vi "TDC_DAQV_CountingRate_muon.vi"(7 "bytes to read":i32=1600, 9 "UDP Config":bool=TRUE, 10 "timeout":dbl=4500.0) -> (0 "error out":errorcluster, 1 "pmt_trigger_rate":dbl[](array[numeric])=[10.0, 4.0, 3.0, 6.0, 13.0, 7.0, 32615.0, 19574.0, 42.0, 11.0, 6.0, 40.0, 20.0, 5.0, 17.0, 21.0, 8.0, 5054.0, 15.0, 837.0, 5.0, 12.0, 0.0, 30.0, 23040.0, 1.0, 7.0, 57773.0, 4.0, 6.0, 15.0, 10.0, 7.0, 2.0, 7.0, 25615.0, 32.0, 54486.0, 5.0, 6.0, 2716.0, 28.0, 4.0, 8.0, 17.0, 17605.0, 8.0, 5695.0, 6.0, 0.0], 2 "time":dbl=450.0011610984802, 3 "rate":dbl=26781.661574353802)   [LabVIEW 2017]
panel:
  out "无符号字节数组":u8[](array[numeric])
  out "Out 2":u8 format="%.0x"
  in  "Array":string[](array[string])=["192.168.10.20"]
  in  "Thresholds":dbl=-0.03
  in  "one key for threshold":bool=TRUE
  out "DAC":dbl=8094.0
  in  "SMA mode":bool
  in  "Thresholds (mV)":dbl[](array[numeric])=[580.0, 580.0, 580.0, 580.0, 600.0, 600.0, 600.0, 600.0, 580.0, 580.0, 600.0, 600.0, 600.0, 600.0, 600.0, 600.0, 580.0, 580.0, 600.0, 600.0, 600.0, 600.0, 600.0, 600.0, 580.0, 580.0, 600.0, 600.0, 600.0, 600.0, 600.0, 600.0, 600.0, 600.0, 600.0, 600.0, 600.0, 600.0, 600.0, 600.0, 600.0, 600.0, 600.0, 600.0, 600.0, 600.0, 600.0, 600.0, 600.0, 600.0, 600.0, 600.0, 600.0, 600.0, 600.0, 600.0, 600.0, 600.0, 600.0, 600.0, 600.0, 600.0, 600.0, 600.0]
  out "Out":u8=3 format="%.0x"
  in  "error in (no error)":errorcluster
  out "rate_array 2":dbl[](array[numeric])=[10.0, 0.0, 4.0, 0.0, 3.0, 0.0, 6.0, 0.0, 13.0, 0.0, 7.0, 0.0, 32615.0, 0.0, 19574.0, 0.0, 42.0, 0.0, 11.0, 0.0, 6.0, 0.0, 40.0, 0.0, 20.0, 0.0, 5.0, 0.0, 17.0, 0.0, 21.0, 0.0, 8.0, 0.0, 5054.0, 0.0, 15.0, 0.0, 837.0, 0.0, 5.0, 0.0, 12.0, 0.0, 0.0, 0.0, 30.0, 0.0, 23040.0, 23040.0, 1.0, 0.0, 7.0, 0.0, 57773.0, 0.0, 4.0, 0.0, 6.0, 0.0, 15.0, 0.0, 10.0, 0.0, 7.0, 0.0, 2.0, 0.0, 7.0, 0.0, 25615.0, 0.0, 32.0, 0.0, 54486.0, 0.0, 5.0, 0.0, 6.0, 0.0, 2716.0, 0.0, 28.0, 0.0, 4.0, 0.0, 8.0, 0.0, 17.0, 0.0, 17605.0, 0.0, 8.0, 0.0, 5695.0, 0.0, 6.0, 0.0, 0.0, 0.0]
  out "数值":dbl=50.0
  out "sent number 2":u64=19574 format="%x"
  out "data 9":string
  out "sent number":u64=3660 format="%x"
  out "substring 2":string
  out "channel number":u64=14 format="%x"
  out "substring":string
  out "array":dbl[](array[numeric])=[-1.0, -1.0, -1.0, -1.0, -1.0, -1.0, -1.0, -1.0, -1.0, -1.0, -1.0, -1.0, -1.0, -1.0, -1.0, -1.0, -1.0, -1.0, -1.0, -1.0, -1.0, -1.0, -1.0, -1.0, -1.0, -1.0, -1.0, -1.0, -1.0, -1.0, -1.0, -1.0, -1.0, -1.0, -1.0, -1.0, -1.0, -1.0, -1.0, -1.0, -1.0, -1.0, -1.0, -1.0, -1.0, -1.0, -1.0, -1.0, -1.0, -1.0, -1.0, -1.0, -1.0, -1.0, -1.0, -1.0, -1.0, -1.0, -1.0, -1.0, -1.0, -1.0, -1.0, -1.0, -1.0, -1.0, -1.0, -1.0, -1.0, -1.0, -1.0, -1.0, -1.0, -1.0, -1.0, -1.0, -1.0, -1.0, -1.0, -1.0, -1.0, -1.0, -1.0, -1.0, -1.0, -1.0, -1.0, -1.0, -1.0, -1.0, -1.0, -1.0, -1.0, -1.0, -1.0, -1.0, -1.0, -1.0, -1.0, -1.0]
  out "trigger number":u64=19574 format="%x"
  out "data 8":string="Lv"
  out "concatenated string":string
  out "number":u32=20
  in  "factor":i32=2
  in  "stop":bool
  in  "timeout (ms)":i32=8400
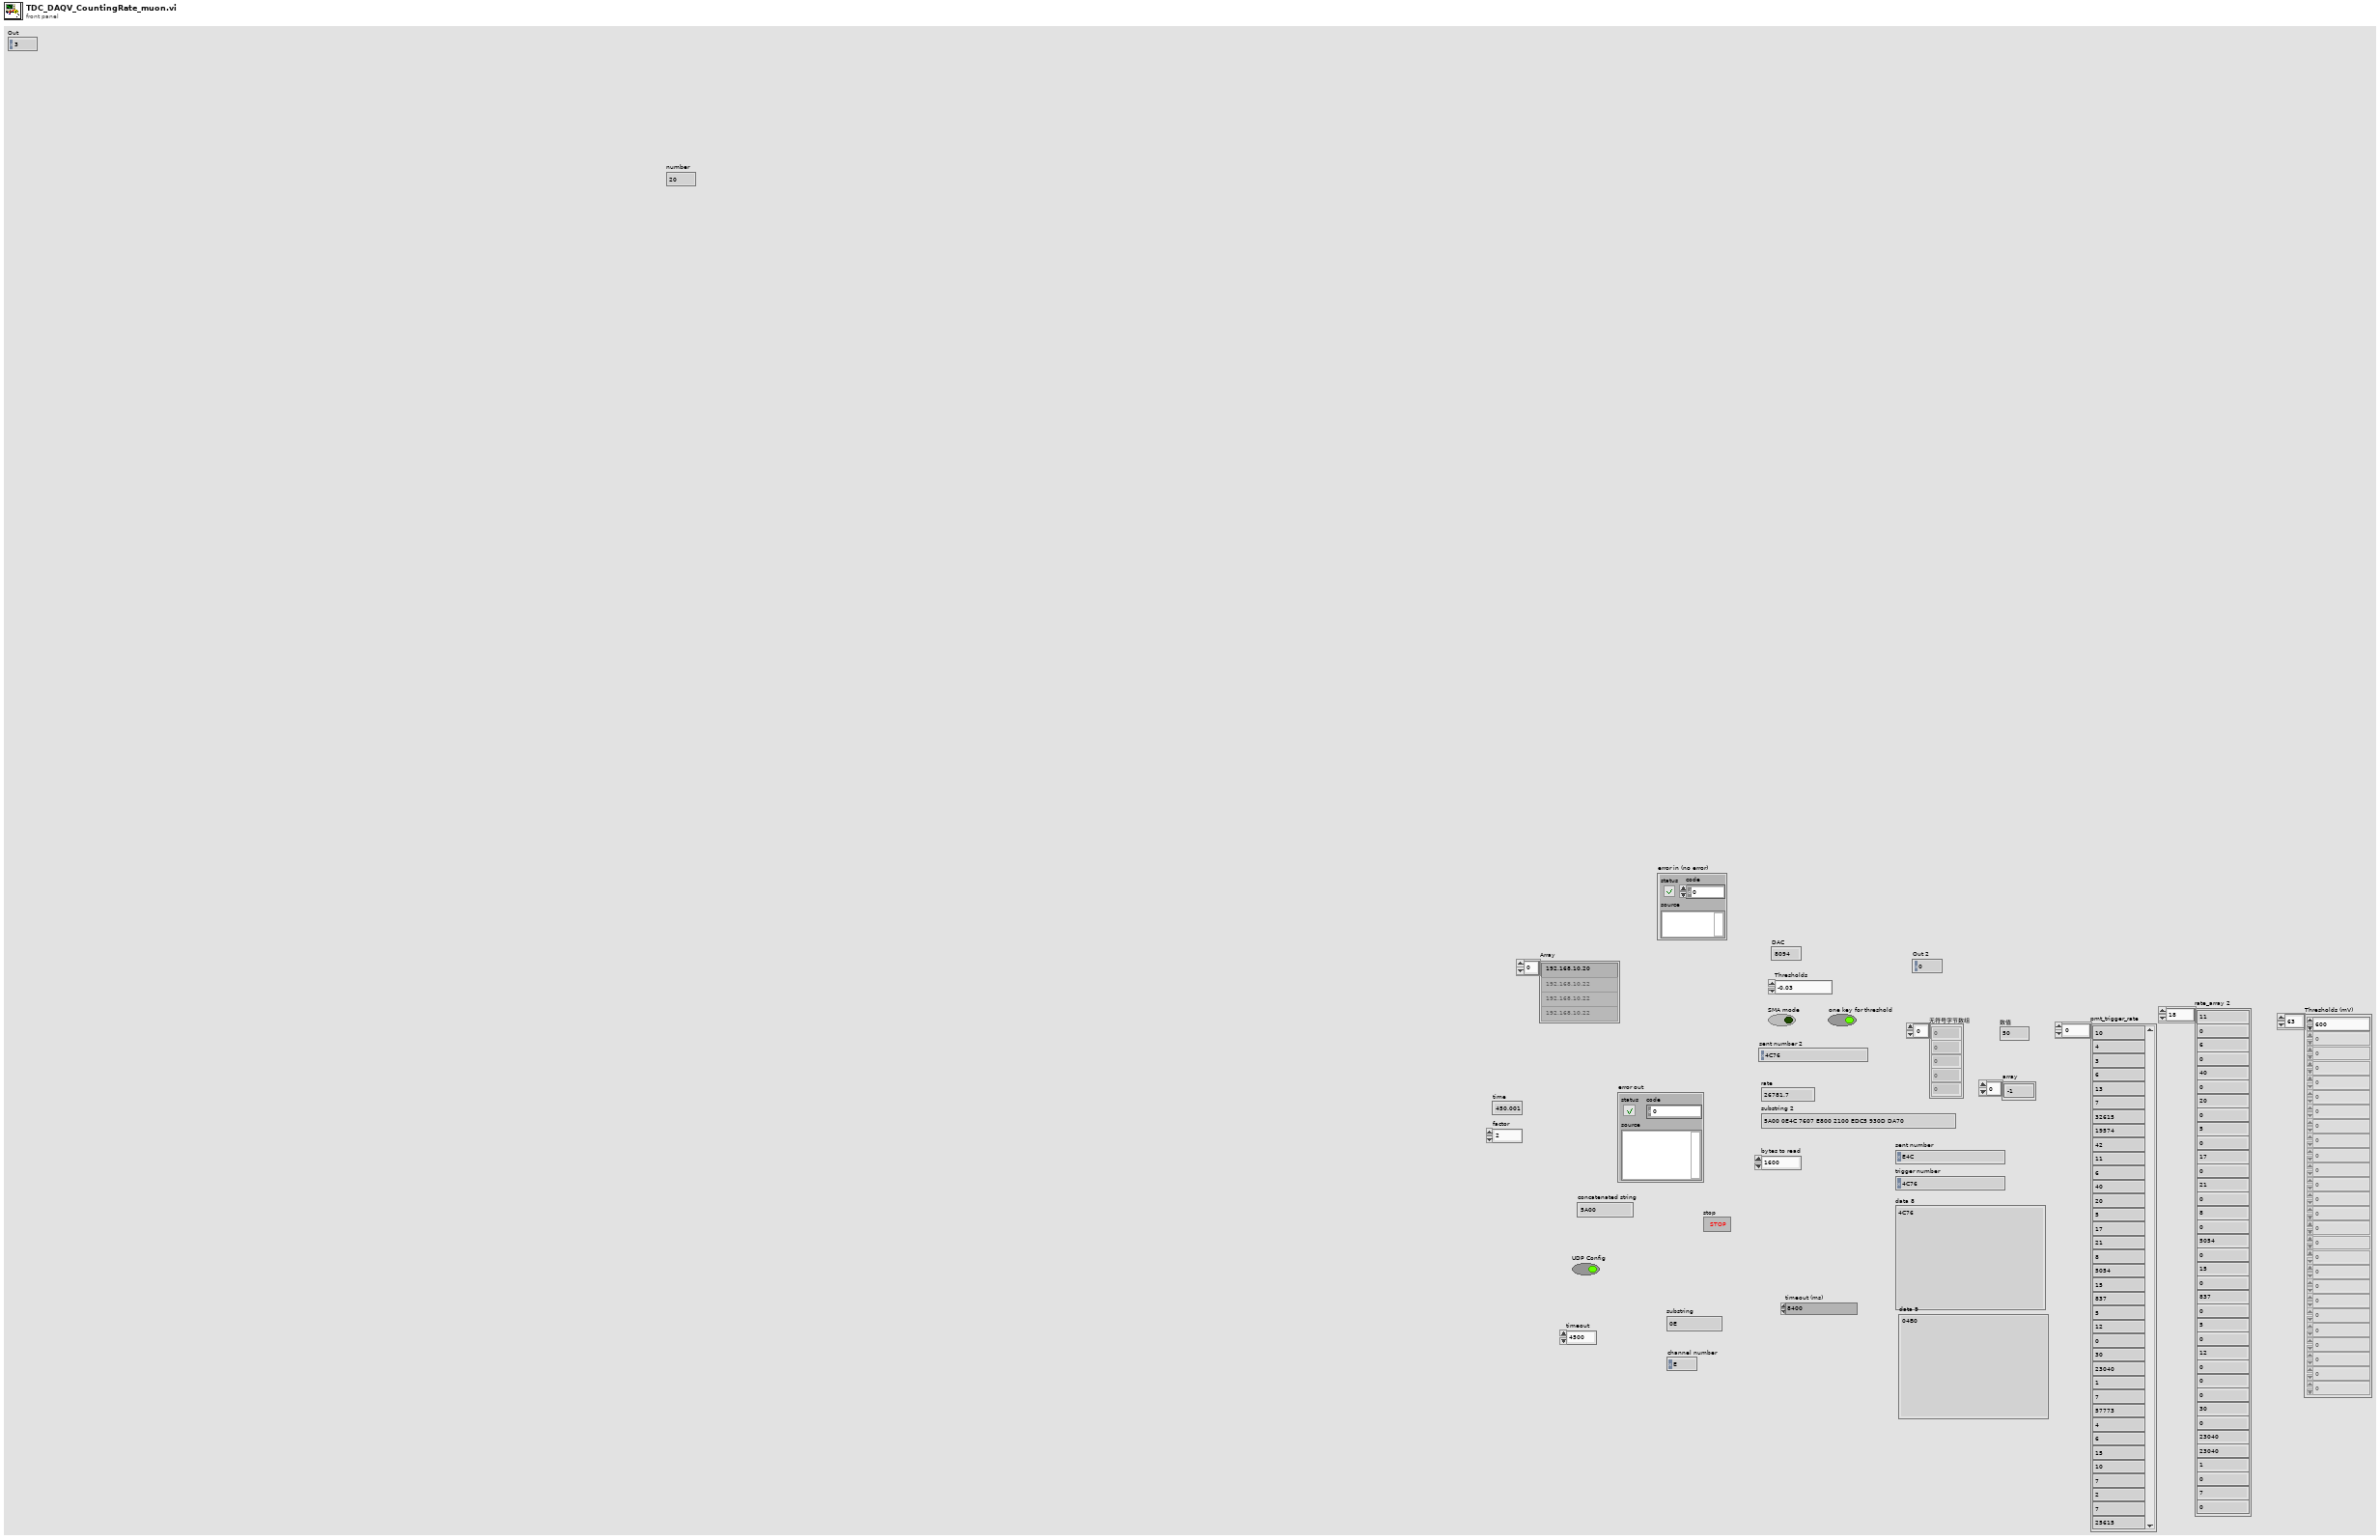
[diagram p1: front panel]
types:
  T1 = enum16{"Standard", "Buffered", "CRLF", "Immediate"}
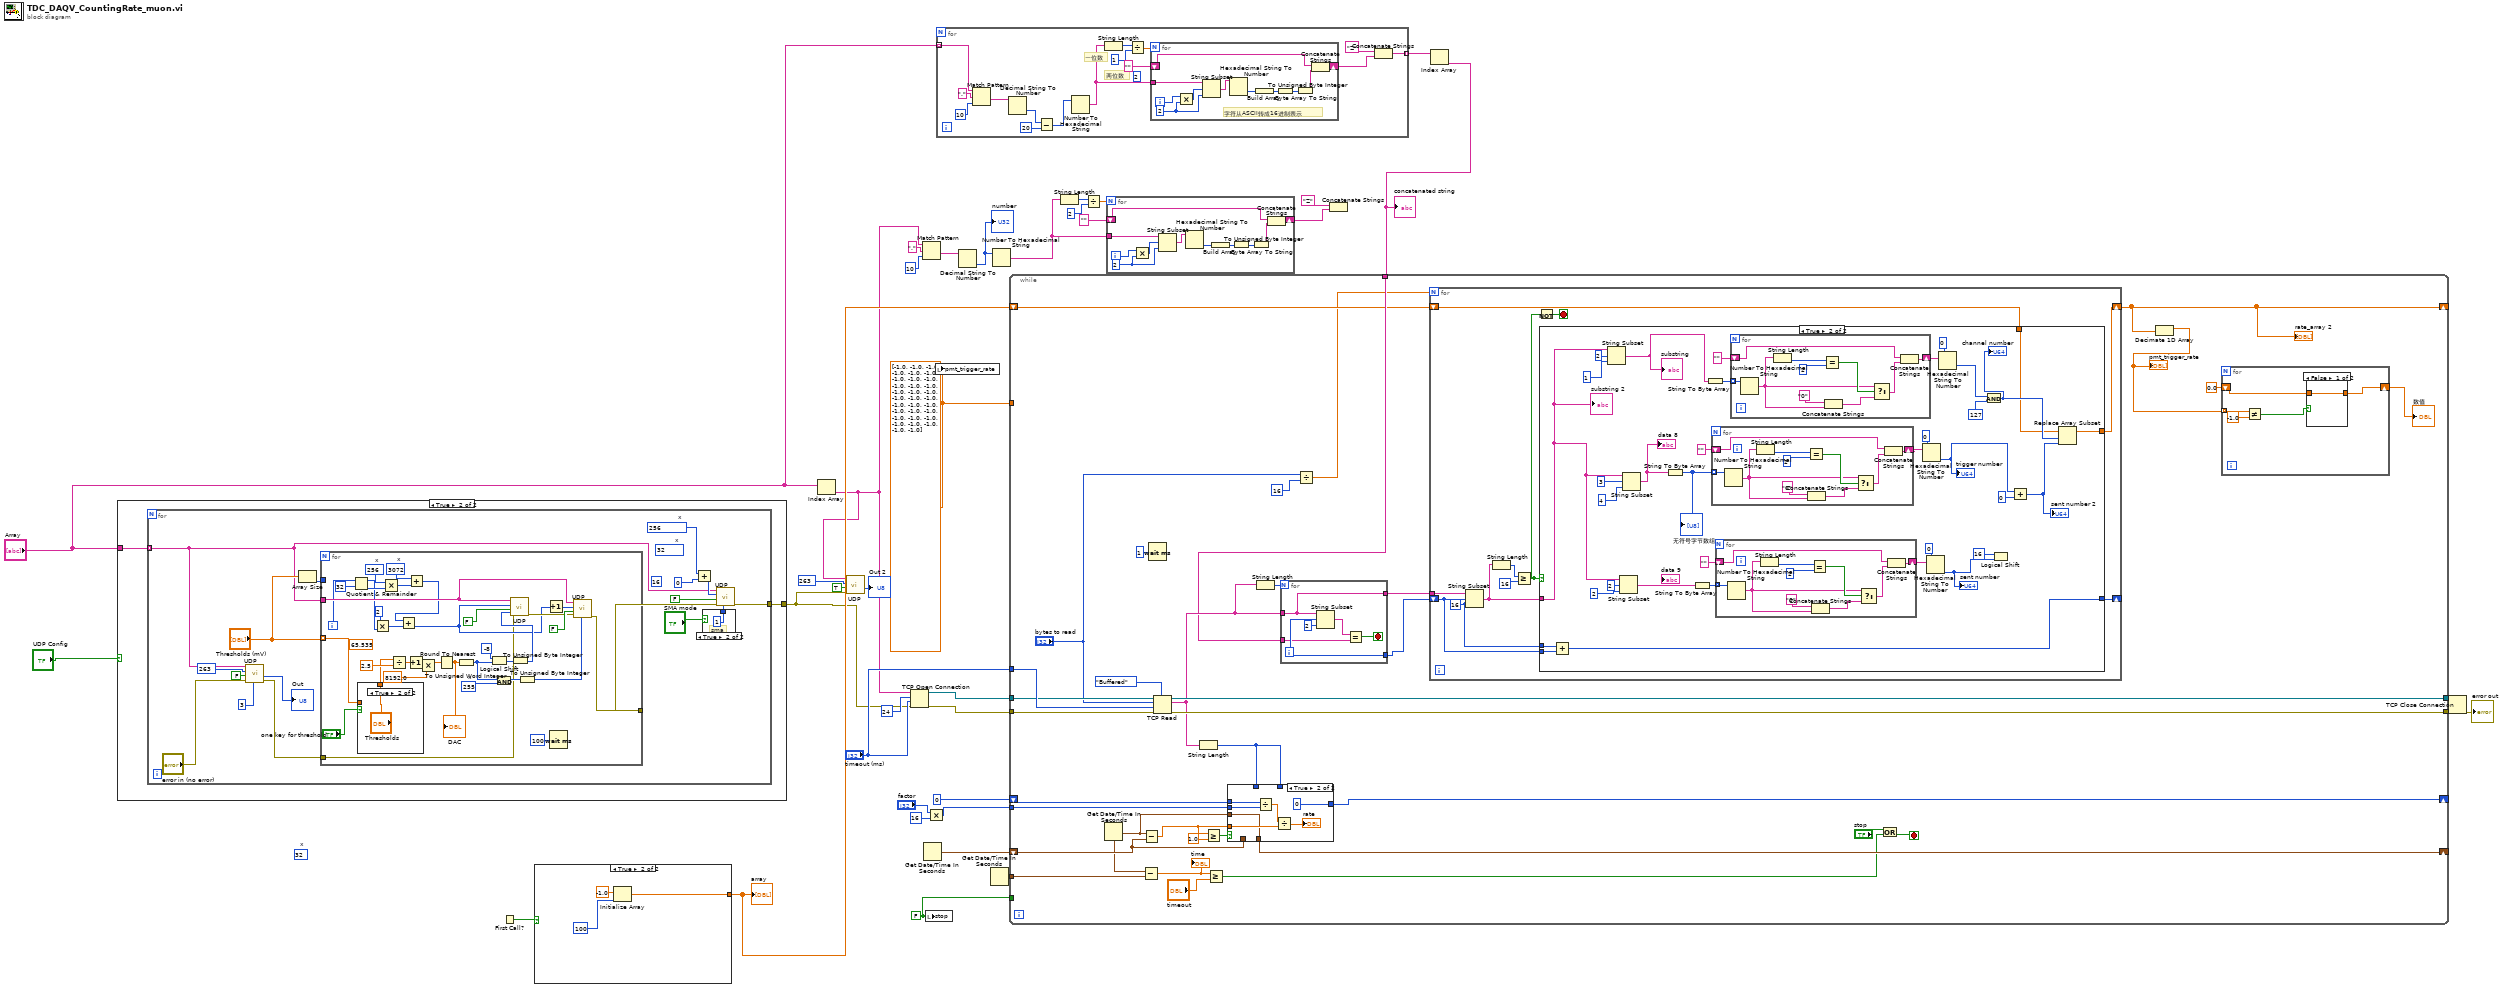
[diagram p0: block diagram]
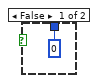
[diagram p3: hidden frame]
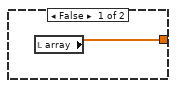
[diagram p5: hidden frame]
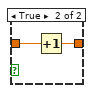
[diagram p6: hidden frame]
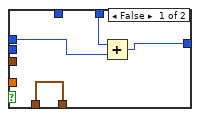
[diagram p8: hidden frame]
diagram:
  w10 = dbl[] [-1.0, -1.0, -1.0, -1.0, -1.0, -1.0, -1.0, -1.0, -1.0, -1.0, -1.0, -1.0, -1.0, -1.0, -1.0, -1.0, -1.0, -1.0, -1.0, -1.0, -1.0, -1.0, -1.0, -1.0, -1.0, -1.0, -1.0, -1.0, -1.0, -1.0, -1.0, -1.0] ("rate_array")
  w25 = FALSE ("stop")
  (unwired) u16 32  # x
  n1 = case shown="True" "UDP Config" {
    tunnel: "Array" -> [_ w38]
    tunnel: [_ w39] -> w3
    frame False {
    }
    frame True {
      n2 = for {
        tunnel: [w54] -> w39
        tunnel: w38 -> [w42] mode=indexing
        (unwired) u16 32  # x
        (unwired) u32 16 ("Address")
        w47 = u16 256  # x
        n3 = call "UDP.vi"("In"=u8 3, "error in (no error)"="error in (no error)", "Read (TRUE)"=FALSE, "Address"=u32 263, "IP address"=w42) -> ("error out"=w40:errorcluster, "Out"=→"Out":u8)  [unwired: 3 in, 1 out]
        n4 = Array Size(array="Thresholds (mV)") -> (size(s)=w51:i32)
        n5 = for {
          tunnel: w42 -> [w88]
          tunnel: "Thresholds (mV)" -> [w75] mode=indexing
          tunnel: [w78] -> w55
          tunnel: w51 -> [_]
          tunnel: w40 -> [w62]
          i -> [w70]
          (unwired) 65.535 ("y")
          w71 = u16 3072  # x
          w72 = u16 256  # x
          w84 = u16 255  # x
          n6 = Quotient & Remainder(x=w70, y=32) -> (x-y*floor(x/y)=w64:i32, floor(x/y)=w73:i32)
          n7 = case shown="True" "one key for threshold" {
            tunnel: [w94 "Thresholds"] -> w76
            tunnel: w75 -> [w94 _]
            frame False {
            }
            frame True {
            }
          }
          n8 = Multiply(x=2, y=w64) -> (x*y=w65:i32)
          n9 = Multiply(x=w72, y=w73) -> (x*y=w67:i32)
          n10 = Divide(x=w76, y=2.5) -> (x/y=w91:dbl)
          n11 = Increment(x=w91) -> (x+1=w61:dbl)
          n12 = Add(x=w71, y=w67) -> (x+y=w66:i32)
          n13 = Add(x=w66, y=w65) -> (x+y=w69:i32)
          n14 = Multiply(x=w61, y=8192.0) -> (x*y=w60:dbl)
          n15 = Round To Nearest(number=w60) -> (nearest integer value=w89:dbl)
          "DAC" <- w89
          n16 = To Unsigned Word Integer(number=w89) -> (unsigned 16bit integer=w80:u16)
          n17 = Logical Shift(y=i16 -8, x=w80) -> (x << y=w86:u16)
          n18 = And(x=w80, y=w84) -> (x .and. y?=w83:u16)
          n19 = To Unsigned Byte Integer(number=w86) -> (unsigned 8bit integer=w85:u8)
          n20 = call "UDP.vi"("In"=w85, "error in (no error)"=w62, "Read (TRUE)"=FALSE, "Address"=w69, "IP address"=w88) -> ("error out"=w79:errorcluster)  [unwired: 3 in, 2 out]
          n21 = To Unsigned Byte Integer(number=w83) -> (unsigned 8bit integer=w82:u8)
          n22 = Increment(x=w69) -> (x+1=w68:i32)
          n23 = Wait (ms)(milliseconds to wait=u32 100) -> ()  [unwired: 1 out]
          n24 = call "UDP.vi"("In"=w82, "error in (no error)"=w79, "Read (TRUE)"=FALSE, "Address"=w68, "IP address"=w88) -> ("error out"=w78:errorcluster)  [unwired: 3 in, 2 out]
        }
        n25 = Add(x=w47, y=u32 0 ("Address")) -> (x+y=w48:u32)
        n26 = case shown="True" "SMA mode" {
          tunnel: [u8 0 ("In") u8 1 ("In")] -> w53
          frame False {
          }
          frame True {
            # "sma"
          }
        }
        n27 = call "UDP.vi"("In"=w53, "error in (no error)"=w55, "Read (TRUE)"=FALSE, "Address"=w48, "IP address"=w42) -> ("error out"=w54:errorcluster)  [unwired: 3 in, 2 out]
      }
    }
  }
  n28 = First Call?() -> (First Call?: T/F=w12:bool)
  n29 = case shown="True" w12 {
    tunnel: [w96 w97] -> w11
    frame False {
      n30 = local read "array"() -> (w96:dbl[])
    }
    frame True {
      n31 = Initialize Array(-1.0 ("element"), 100 ("dimension size")) -> (w97:dbl[])
    }
  }
  "array" <- w11
  n32 = Index Array(array="Array") -> (element=w2:string)  [unwired: 1 in]
  n33 = call "UDP.vi"("error in (no error)"=w3, "Read (TRUE)"=TRUE, "Address"=u32 263, "IP address"=w2) -> ("Out"=→"Out 2":u8)  [unwired: 4 in, 2 out]
  n34 = TCP Open Connection(address=w2, remote port or service name=u16 24 ("port"), timeout ms (60000)="timeout (ms)", error in (no error)=w3) -> (connection ID=w35:refnum<k5>, error out=w36:errorcluster)  [unwired: 1 in]
  n35 = Match Pattern(string=w2, regular expression="." ("search string"), offset (0)=10) -> (after substring=w16:string)  [unwired: 3 out]
  n36 = Get Date/Time In Seconds() -> (seconds since 1Jan1904=w31:timestamp)
  n37 = local write "stop"(w25) -> ()
  n38 = Multiply(x="factor", y=16) -> (x*y=w27:i32)
  n39 = local write "pmt_trigger_rate"(w10) -> ()
  n40 = for {
    tunnel: [w101] -> w7 mode=indexing
    tunnel: "Array" -> [w100] mode=indexing
    (unwired) 2 ("y")
    # "一位数"
    # "两位数"
    n41 = Match Pattern(string=w100, regular expression="." ("search string"), offset (0)=10) -> (after substring=w107:string)  [unwired: 3 out]
    n42 = Decimal String To Number(string=w107) -> (number=w104:i32)  [unwired: 2 in, 1 out]
    n43 = Subtract(x=w104, y=20) -> (x-y=w103:i32)
    n44 = Number To Hexadecimal String(2:w103) -> (0:w106:string)  [unwired: 1 in]
    n45 = String Length(string=w106) -> (length=w112:i32)
    n46 = Divide(x=w112, y=1) -> (x/y=w113:dbl)
    n47 = for {
      N: w113 -> [_]
      shift-right: [w125] -> w102
      shift-left: "" ("format string") -> [w124]
      tunnel: w106 -> [w115]
      i -> [w123]
      w117 = 2 ("y")
      # "字符从ASCII转成16进制表示"
      n48 = Multiply(x=w123, y=w117) -> (x*y=w116:i32)
      n49 = String Subset(string=w115, offset (0)=w116, length (rest)=w117) -> (substring=w118:string)
      n50 = Hexadecimal String To Number(string=w118) -> (number=w122:u32)  [unwired: 2 in, 1 out]
      n51 = Build Array(w122) -> (w121:u32[])
      n52 = To Unsigned Byte Integer(number=w121) -> (unsigned 8bit integer=w120:u8[])
      n53 = Byte Array To String(unsigned byte array=w120) -> (string=w119:string)
      n54 = Concatenate Strings(w124, w119) -> (w125:string)
    }
    n55 = Concatenate Strings("Z", w102) -> (w101:string)
  }
  n56 = Decimal String To Number(string=w16) -> (number=w15:i32)  [unwired: 2 in, 1 out]
  "number" <- w15
  n57 = Get Date/Time In Seconds() -> (seconds since 1Jan1904=w24:timestamp)
  n58 = Number To Hexadecimal String(2:w15) -> (0:w14:string)  [unwired: 1 in]
  n59 = String Length(string=w14) -> (length=w21:i32)
  n60 = Divide(x=w21, y=2) -> (x/y=w22:dbl)
  n61 = for {
    N: w22 -> [_]
    shift-right: [w136] -> w13
    shift-left: "" ("format string") -> [w135]
    tunnel: w14 -> [w126]
    i -> [w134]
    w128 = 2 ("y")
    n62 = Multiply(x=w134, y=w128) -> (x*y=w127:i32)
    n63 = String Subset(string=w126, offset (0)=w127, length (rest)=w128) -> (substring=w129:string)
    n64 = Hexadecimal String To Number(string=w129) -> (number=w133:u32)  [unwired: 2 in, 1 out]
    n65 = Build Array(w133) -> (w132:u32[])
    n66 = To Unsigned Byte Integer(number=w132) -> (unsigned 8bit integer=w131:u8[])
    n67 = Byte Array To String(unsigned byte array=w131) -> (string=w130:string)
    n68 = Concatenate Strings(w135, w130) -> (w136:string)
  }
  n69 = Concatenate Strings("Z", w13) -> ()  [unwired: 1 out]
  n70 = Index Array(array=w7) -> (element=w6:string)  [unwired: 1 in]
  "concatenated string" <- w6
  n71 = while {
    tunnel: w36 -> [w172]
    tunnel: "timeout (ms)" -> [w171]
    tunnel: w35 -> [w170]
    tunnel: [w169] -> w34
    tunnel: [w168] -> w33
    shift-right: [w161] -> _
    shift-left: w31 -> [w165]
    shift-right: [w164] -> _
    shift-left: u32 0 ("milliseconds to wait") -> [w159]
    tunnel: w27 -> [w158]
    tunnel: w25 -> [_]
    tunnel: w24 -> [w152]
    tunnel: w6 -> [w146]
    shift-right: [w137] -> _
    shift-left: w11 -> [w145]
    tunnel: w10 -> [_]
    stop <- w155 stop-if-true
    n72 = Get Date/Time In Seconds() -> (seconds since 1Jan1904=w151:timestamp)
    n73 = Subtract(x=w151, y=w152) -> (x-y=w150:dbl)
    "time" <- w150
    n74 = Subtract(x=w151, y=w165) -> (x-y=w157:dbl)
    n75 = Wait (ms)(milliseconds to wait=u32 1) -> ()  [unwired: 1 out]
    n76 = TCP Read(connection ID=w170, bytes to read="bytes to read", error in (no error)=w172, 7:T1."Buffered" ("mode (standard)"), 9:w171) -> (connection ID out=w169:refnum<k5>, data out=w147:string, error out=w168:errorcluster)
    n77 = String Length(string=w147) -> (length=w160:i32)
    n78 = Greater Or Equal?(x=w157, y=1.0) -> (x >= y?=w163:bool)
    n79 = Greater Or Equal?(x=w150, y="timeout") -> (x >= y?=w153:bool)
    n80 = case shown="True" w163 {
      tunnel: w157 -> [_ w275]
      tunnel: w151 -> [_ w273]
      tunnel: [w268 w273] -> w161
      tunnel: w165 -> [w268 _]
      tunnel: w160 -> [_ _]
      tunnel: w160 -> [w267 _]
      tunnel: [w266 0] -> w164
      tunnel: w158 -> [_ w270]
      tunnel: w159 -> [w265 w269]
      frame False {
        n81 = Add(x=w267, y=w265) -> (x+y=w266:u32)
      }
      frame True {
        n82 = Divide(x=w269, y=w270) -> (x/y=w272:dbl)
        n83 = Divide(x=w272, y=w275) -> (x/y=→"rate":dbl)
      }
    }
    n84 = String Length(string=w147) -> (length=w149:i32)
    n85 = for {
      N: w149 -> [_]
      tunnel: w147 -> [w261]
      tunnel: [w261] -> w148
      tunnel: [w260] -> w144
      tunnel: w146 -> [w259]
      i -> [w260]
      stop <- w262 stop-if-true
      n86 = String Subset(string=w261, offset (0)=w260, length (rest)=2 ("length (rest)")) -> (substring=w263:string)
      n87 = Equal?(x=w263, y=w259) -> (x = y?=w262:bool)
    }
    n88 = Divide(x="bytes to read", y=16 ("length (rest)")) -> (x/y=w141:dbl)
    n89 = for {
      N: w141 -> [_]
      tunnel: w148 -> [w191]
      shift-right: [w189] -> w137
      shift-left: w145 -> [w190]
      shift-right: [w181] -> _
      shift-left: w144 -> [w182]
      stop <- w184 stop-if-true
      w183 = 16 ("length (rest)")
      n90 = String Subset(string=w191, offset (0)=w182, length (rest)=w183) -> (substring=w188:string)
      n91 = String Length(string=w188) -> (length=w187:i32)
      n92 = Greater Or Equal?(x=w187, y=16 ("length (rest)")) -> (x >= y?=w185:bool)
      n93 = Not(x=w185) -> (.not. x?=w184:bool)
      n94 = case shown="True" w185 {
        tunnel: w188 -> [_ w209]
        tunnel: w190 -> [w193 w208]
        tunnel: [w193 w207] -> w189
        tunnel: w182 -> [w192 w206]
        tunnel: w183 -> [_ w205]
        tunnel: [w192 w204] -> w181
        frame False {
        }
        frame True {
          n95 = Add(x=w205, y=w206) -> (x+y=w204:i32)
          n96 = String Subset(string=w209, offset (0)=2, length (rest)=1 ("length (rest)")) -> (substring=w213:string)
          "substring" <- w213
          n97 = String Subset(string=w209, offset (0)=2, length (rest)=2 ("length (rest)")) -> (substring=w199:string)
          n98 = String Subset(string=w209, offset (0)=3, length (rest)=4 ("length (rest)")) -> (substring=w220:string)
          "data 8" <- w220
          n99 = String To Byte Array(string=w220) -> (unsigned byte array=w222:u8[])
          "无符号字节数组" <- w222
          n100 = String To Byte Array(string=w199) -> (unsigned byte array=w202:u8[])
          n101 = String To Byte Array(string=w213) -> (unsigned byte array=w216:u8[])
          n102 = for {
            shift-right: [w257] -> w223
            shift-left: "" ("format string") -> [w254]
            tunnel: w222 -> [w258] mode=indexing
            n103 = Number To Hexadecimal String(2:w258) -> (0:w250:string)  [unwired: 1 in]
            n104 = String Length(string=w250) -> (length=w256:i32)
            n105 = Equal?(x=w256, y=2) -> (x = y?=w253:bool)
            n106 = Concatenate Strings("0" ("format string"), w250) -> (w252:string)
            n107 = Select(t=w250, s=w253, f=w252) -> (s? t:f=w249:string)
            n108 = Concatenate Strings(w254, w249) -> (w257:string)
          }
          n109 = for {
            shift-right: [w237] -> w201
            shift-left: "" ("format string") -> [w234]
            tunnel: w202 -> [w238] mode=indexing
            n110 = Number To Hexadecimal String(2:w238) -> (0:w230:string)  [unwired: 1 in]
            n111 = String Length(string=w230) -> (length=w236:i32)
            n112 = Equal?(x=w236, y=2) -> (x = y?=w233:bool)
            n113 = Concatenate Strings("0" ("format string"), w230) -> (w232:string)
            n114 = Select(t=w230, s=w233, f=w232) -> (s? t:f=w229:string)
            n115 = Concatenate Strings(w234, w229) -> (w237:string)
          }
          n116 = for {
            shift-right: [w247] -> w215
            shift-left: "" ("format string") -> [w244]
            tunnel: w216 -> [w248] mode=indexing
            n117 = Number To Hexadecimal String(2:w248) -> (0:w240:string)  [unwired: 1 in]
            n118 = String Length(string=w240) -> (length=w246:i32)
            n119 = Equal?(x=w246, y=2) -> (x = y?=w243:bool)
            n120 = Concatenate Strings("0" ("format string"), w240) -> (w242:string)
            n121 = Select(t=w240, s=w243, f=w242) -> (s? t:f=w239:string)
            n122 = Concatenate Strings(w244, w239) -> (w247:string)
          }
          n123 = Hexadecimal String To Number(string=w223, default (0uL)=u64 0 ("default (0 U32)")) -> (number=w196:u64)  [unwired: 1 in, 1 out]
          "trigger number" <- w196
          n124 = Hexadecimal String To Number(string=w201, default (0uL)=u64 0 ("default (0 U32)")) -> (number=w198:u64)  [unwired: 1 in, 1 out]
          "sent number" <- w198
          n125 = Hexadecimal String To Number(string=w215, default (0uL)=u64 0 ("default (0 U32)")) -> (number=w212:u64)  [unwired: 1 in, 1 out]
          n126 = And(x=w212, y=u64 127 ("default (0 U32)")) -> (x .and. y?=w210:u64)
          "channel number" <- w210
          n127 = Logical Shift(y=i16 16, x=w198) -> ()  [unwired: 1 out]
          n128 = Add(x=w196, y=u64 0) -> (x+y=w195:u64)
          "sent number 2" <- w195
          n129 = Replace Array Subset(array=w208, new element=w195, index=w210) -> (w207:dbl[])
          "substring 2" <- w209
        }
      }
    }
    "rate_array 2" <- w137
    n130 = Or(x="stop", y=w153) -> (x .or. y?=w155:bool)
    n131 = Decimate 1D Array(w137) -> (w140:dbl[])  [unwired: 1 out]
    "pmt_trigger_rate" <- w140
    n132 = for {
      tunnel: w140 -> [w177] mode=indexing
      shift-right: [w173] -> w138
      shift-left: 0.0 -> [w174]
      n133 = Not Equal?(x=w177, y=-1.0) -> (x != y?=w175:bool)
      n134 = case shown="False" w175 {
        tunnel: w174 -> [w178 w180]
        tunnel: [w178 w179] -> w173
        frame False {
        }
        frame True {
          n135 = Increment(x=w180) -> (x+1=w179:dbl)
        }
      }
    }
    "数值" <- w138
  }
  n136 = TCP Close Connection(connection ID=w34, error in (no error)=w33) -> (error out=→"error out":errorcluster)  [unwired: 1 in, 1 out]
